vi "DAQ AI Inventory (SubVI).vi"(8 "error in (no error)":errorcluster, 10 "DAQ AI address":tag[](array[tag]), 11 "Use DAQ AI?":bool[](array[boolean])) -> (0 "error out":errorcluster, 1 "present values out":dbl[](array[numeric]), 2 "DAQ AI Address out":refnum<k21>[](array[refnum]), 3 "DAQ names out":string[](array[string]))   [LabVIEW 2025, in "MyDaq.lvlib"]
uses:
  MyDaq.lvlib
  <vilib>/DAQmx/read.llb/DAQmx Read (Analog DBL 1Chan 1Samp).vi
  <vilib>/DAQmx/create/channels.llb/DAQmx Create Channel (AI-Voltage-Basic).vi
  <vilib>/DAQmx/miscellaneous.llb/DAQmx Fill In Error Info.vi
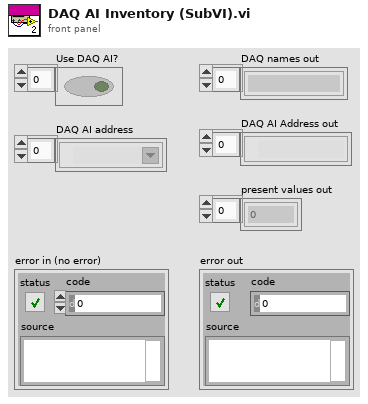
[diagram p1: front panel]
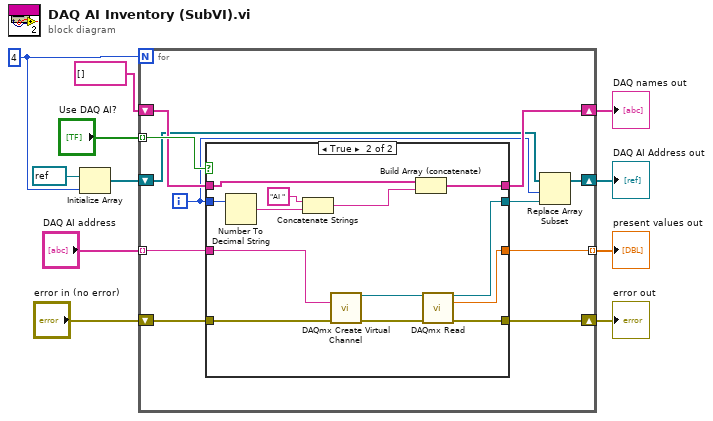
[diagram p0: block diagram]
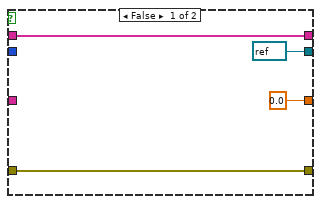
[diagram p2: hidden frame]
diagram:
  w5 = 4
  n1 = Initialize Array(refnum<k21> refnum ("task out"), w5) -> (w3:refnum<k21>[])
  n2 = for {
    N: w5 -> [_]
    shift-right: [w21] -> w7
    shift-left: "error in (no error)" -> [w22]
    tunnel: "Use DAQ AI?" -> [w20] mode=indexing
    tunnel: "DAQ AI address" -> [w17] mode=indexing
    tunnel: [w16] -> w11 mode=indexing
    shift-right: [w13] -> w2
    shift-left: w3 -> [w15]
    shift-right: [w19] -> w8
    shift-left: string[] [] ("DAQ names in") -> [w18]
    i -> [w12]
    n3 = case shown="True" w20 {
      tunnel: w17 -> [_ w37]
      tunnel: [refnum<k21> refnum ("task out") w36] -> w14
      tunnel: w22 -> [w26 w35]
      tunnel: [w26 w34] -> w21
      tunnel: [w23 w31] -> w19
      tunnel: w18 -> [w23 w32]
      tunnel: [0.0 ("data") w33] -> w16
      tunnel: w12 -> [_ w27]
      frame False {
      }
      frame True {
        n4 = Number To Decimal String(number=w27) -> (decimal integer string=w29:string)  [unwired: 1 in]
        n5 = Concatenate Strings("AI " ("string"), w29) -> (w28:string)
        n6 = call-poly <vilib>:"DAQmx Create Virtual Channel.vi"("physical channels"=w37, "error in"=w35) -> ("task out"=w39:refnum<k21>, "error out"=w38:errorcluster)  [unwired: 12 in]
        n7 = Build Array (concatenate)(w32, w28) -> (w31:string[])
        n8 = call-poly <vilib>:"DAQmx Read.vi"("task/channels in"=w39, "error in"=w38) -> ("task out"=w36:refnum<k21>, "data"=w33:dbl, "error out"=w34:errorcluster)  [unwired: 11 in]
      }
    }
    n9 = Replace Array Subset(array=w15, new element=w14, index=w12) -> (w13:refnum<k21>[])
  }
  "present values out" <- w11
  "DAQ names out" <- w8
  "DAQ AI Address out" <- w2
  "error out" <- w7
